vi "Create by Ref.vi"(0 "error in (no error)":errorcluster caption="错误输入（无错误）", 3 "StatusStrip":refnum<k24>) -> (7 "error out":errorcluster caption="错误输出", 10 "StatusStripClass 输出":refnum<class "StatusStripClass.lvclass"> caption="DNL_LabVIEW Object out")   [LabVIEW 2013, in "StatusStripClass.lvclass"]
uses:
  StatusStripClass.lvclass
  System.Windows.Forms
  StatusStripClass.lvclass/StatusStripClass.ctl
panel:
  in  "StatusStripClass 输入":refnum<class "StatusStripClass.lvclass"> caption="DNL_LabVIEW Object in"
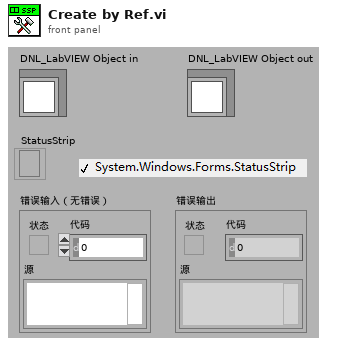
[diagram p1: front panel]
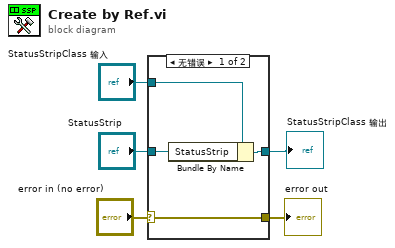
[diagram p0: block diagram]
diagram:
  n1 = case shown="无错误" "error in (no error)" {
    selector: "error in (no error)" -> [w9 w11]
    tunnel: [w9 w11] -> w4
    tunnel: [w7 w10] -> w2
    tunnel: "StatusStripClass 输入" -> [w8 w10]
    tunnel: "StatusStrip" -> [w6 _]
    frame No Error {
      n2 = Bundle By Name(cluster=w8, "StatusStrip"=w6) -> (w7:refnum<class "StatusStripClass.lvclass">)
    }
    frame Error {
    }
  }
  "error out" <- w4
  "StatusStripClass 输出" <- w2
